vi "Create GB.vi"(5 "Max # of atoms":i32=9999999, 6 "Edge Duplication Range":dbl=3.0, 7 "Skip cleanup if no subset":bool=TRUE, 8 "Reduce to Repeating":T5={"Slab X"=4.6, "Slab Y"=4.0, "Tolerance (A)"=0.5, "Presorted?"=FALSE}, 9 "Min Seperation Distance (A)":dbl=2.0, 10 "Grain Growth and Geometry":T6={"Min Grain 1 Length (A)"=6.0, "Min Grain 2 Length (A)"=6.0, "Max Grain Height (A)"=90.0, "Max Grain Width (A)"=90.0, "Grain 1 Start"=-0.001, "Overlap Region (A)"=0.001}, 11 "Grain Boundary Definition":T7={"Grain 1 Orientation"=[1.0, 0.6019417241891012, 0.029651947654046266], "Grain 2 Orientation"=[1.0, 0.730727623275494, 0.2205637301176], "Twist Angle (Deg)"=0.0, "Translation Vector"=[0.0, 0.0, 0.0]}) -> (0 "GB Data":string[][](array[string])=[["Grain 1, h", "Grain 1, k", "Grain 1, L", "Grain 2, h", "Grain 2, k", "Grain 2, L", "Twist Angle (Deg)", "Translation Tx", "Translation Ty", "Translation Tz", "Tilt Angle (Deg)", "Viewing Angle, h", "Viewing Angle, k", "Viewing Angle, L", "Grain 1 Length (factor)", "Grain 2 Length (factor", "Max Grain Height (A)", "Max Grain Width (A)", "Grain 1 Start", "Overlap Region (A)", "Reduction Slab X", "Reduction Slab Y", "Reduction Tolerance (A)", "Min Atomic Separation Distance", "Edge Duplication Range", "# Atoms"], ["1.000000", "0.601942", "0.029652", "1.000000", "0.730728", "0.220564", "0.000000", "0.000000", "0.000000", "0.000000", "10.024930", "1.000000", "-1.661290", "0.000000", "1.000000", "1.000000", "90.000000", "90.000000", "-0.001000", "0.001000", "4.600000", "4.000000", "0.500000", "2.000000", "3.000000", "12135.000000"]], 1 "Reduced Orthorhombic?":bool, 2 "Reduced Rhombahedral?":bool, 3 "Grain Boundary":T8={"Structure Name"="(0.00) twist [1.000,0.602,0.030] [1.000,0.731,0.221] (0.00,0.00,0.00)T GB", "Lattice vector a"=[270.03, 0.0, 0.0], "Lattice vector b"=[0.0, 270.03, 0.0], "Lattice vector c"=[0.0, 0.0, 6.006], "Atoms Array"=[{"Atom Name"="Cd", "Positions (Direct)"=array6055x3[18165 elements], "Positions (Cartesian)"=array6055x3[18165 elements]}, {"Atom Name"="Te", "Positions (Direct)"=array6080x3[18240 elements], "Positions (Cartesian)"=array6080x3[18240 elements]}], "# of atoms"=12135} {"Atoms Array"."Positions (Cartesian)" format="%#_4f"; "Atoms Array"."Positions (Direct)" format="%#_4f"}, 4 "Ortho and Rhom":T3(array[cluster]) {"Atoms Array"."Positions (Cartesian)" format="%#_4f"; "Atoms Array"."Positions (Direct)" format="%#_4f"})   [LabVIEW 2010]
uses:
  <vilib>/Analysis/NI_AALPro.lvlib
  <vilib>/Analysis/_algsub.llb/Real Vector Norm.vi
  <vilib>/Analysis/NI_AALBase.lvlib
  <vilib>/Analysis/baseanly.llb/A x Vector.vi
  <vilib>/Analysis/baseanly.llb/Real A x B.vi
panel:
  in  "GB Reduction":T1(radio)
  in  "GB Geometry":T2(radio)
  in  "Min Wedge Thickness (A)":dbl=5.0
  out "error out":errorcluster
  out "Original # of atoms":i32=12135
  out "Expected # of Atoms":i32=166
  in  "Integer Tolerance":dbl=0.01
  out "Creation Time":T4={"Time to create primitives"=0, "Time to Grow to Box"=4152, "Time to find subset"=1109, "Time to Cleanup"=1}
  in  "Headers":string[](array[string])=["Grain 1, h", "Grain 1, k", "Grain 1, L", "Grain 2, h", "Grain 2, k", "Grain 2, L", "Twist Angle (Deg)", "Translation Tx", "Translation Ty", "Translation Tz", "Tilt Angle (Deg)", "Viewing Angle, h", "Viewing Angle, k", "Viewing Angle, L", "Grain 1 Length (factor)", "Grain 2 Length (factor", "Max Grain Height (A)", "Max Grain Width (A)", "Grain 1 Start", "Overlap Region (A)", "Reduction Slab X", "Reduction Slab Y", "Reduction Tolerance (A)", "Min Atomic Separation Distance", "Edge Duplication Range", "# Atoms"]
  out "Rhombehedral Atoms":i32=12135
  out "Orthorhombic atoms":i32=12135
  out "Time to Cleanup":u32=1
  out "Time to find subset":u32=1109
  out "Time to Grow to Box":u32=4152
  out "Time to create primitives":u32
  out "Tilt Angle":dbl=10.024929742348679
  out "# of Atoms Removed":i32=28
  out "Repeating Y Length Scale":dbl=13.227303403298492
  out "Repeating X Length Scale":dbl
  out "Mutual Viewing Angle":dbl[](array[numeric])=[1.0, -1.6612903871170226, 0.0]
  in  "Conventional Unit Cell":T8={"Structure Name"="CdTe", "Lattice vector a"=[6.615785553057252, 0.0, 0.0], "Lattice vector b"=[0.0, 6.615785553057252, 0.0], "Lattice vector c"=[0.0, 0.0, 6.615785553057252], "Atoms Array"=[{"Atom Name"="Cd", "Positions (Direct)"=[[0.0, 0.0, 0.0], [0.0, 0.5, 0.5], [0.5, 0.0, 0.5], [0.5, 0.5, 0.0]], "Positions (Cartesian)"=[[0.0, 0.0, 0.0], [0.0, 3.307892776528626, 3.307892776528626], [3.307892776528626, 0.0, 3.307892776528626], [3.307892776528626, 3.307892776528626, 0.0]]}, {"Atom Name"="Te", "Positions (Direct)"=[[0.25, 0.25, 0.25], [0.75, 0.75, 0.25], [0.75, 0.25, 0.75], [0.25, 0.75, 0.75]], "Positions (Cartesian)"=[[1.653946388264313, 1.653946388264313, 1.653946388264313], [4.96183916479294, 4.96183916479294, 1.653946388264313], [4.96183916479294, 1.653946388264313, 4.96183916479294], [1.653946388264313, 4.96183916479294, 4.96183916479294]]}], "# of atoms"=8}
  # "Primitives"
  # "Remove Collisions"
  # "Make into repeating cell"
  # "Grain Growth"
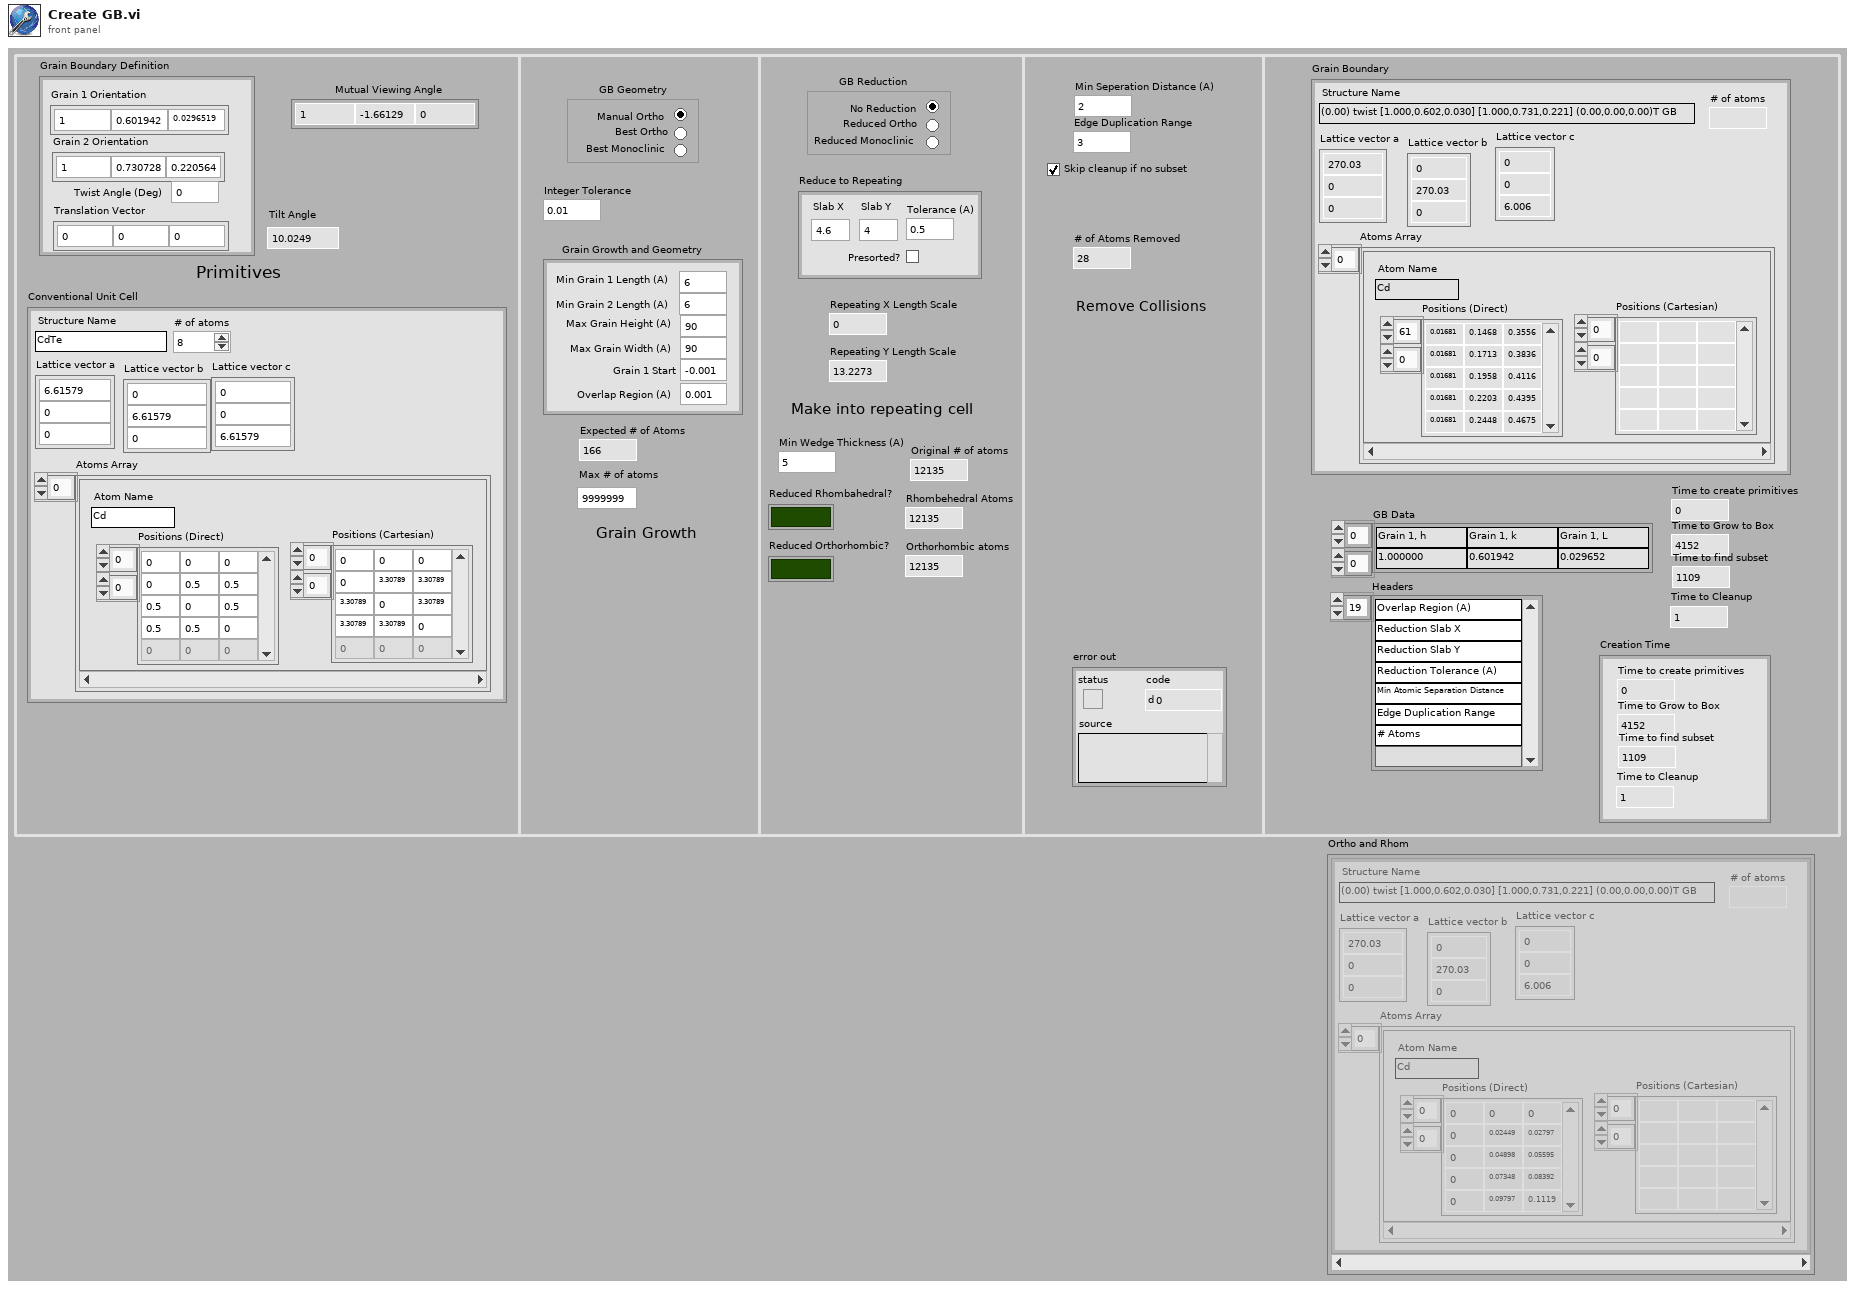
[diagram p1: front panel]
types:
  T1 = enum32{"No Reduction", "Reduced Ortho", "Reduced Monoclinic"}
  T2 = enum32{"Manual Ortho", "Best Ortho", "Best Monoclinic"}
  T3 = cluster{"Structure Name":string, "Lattice vector a":dbl[], "Lattice vector b":dbl[], "Lattice vector c":dbl[], "Atoms Array":cluster{"Atom Name":string, "Positions (Direct)":dbl[][], "Positions (Cartesian)":dbl[][]}[], "# of atoms":i32}[]
  T4 = cluster{"Time to create primitives":u32, "Time to Grow to Box":u32, "Time to find subset":u32, "Time to Cleanup":u32}
  T5 = cluster{"Slab X":dbl, "Slab Y":dbl, "Tolerance (A)":dbl, "Presorted?":bool}
  T6 = cluster{"Min Grain 1 Length (A)":dbl, "Min Grain 2 Length (A)":dbl, "Max Grain Height (A)":dbl, "Max Grain Width (A)":dbl, "Grain 1 Start":dbl, "Overlap Region (A)":dbl}
  T7 = cluster{"Grain 1 Orientation":dbl[], "Grain 2 Orientation":dbl[], "Twist Angle (Deg)":dbl, "Translation Vector":dbl[]}
  T8 = cluster{"Structure Name":string, "Lattice vector a":dbl[], "Lattice vector b":dbl[], "Lattice vector c":dbl[], "Atoms Array":cluster{"Atom Name":string, "Positions (Direct)":dbl[][], "Positions (Cartesian)":dbl[][]}[], "# of atoms":i32}
  T9 = cluster{"Grain 1 Orientation":dbl[], "Grain 2 Orientation":dbl[], "Twist Angle (Deg)":dbl}
  T10 = typedef "NI_Matrix.lvlib/RealMatrix.ctl" = dbl[][]
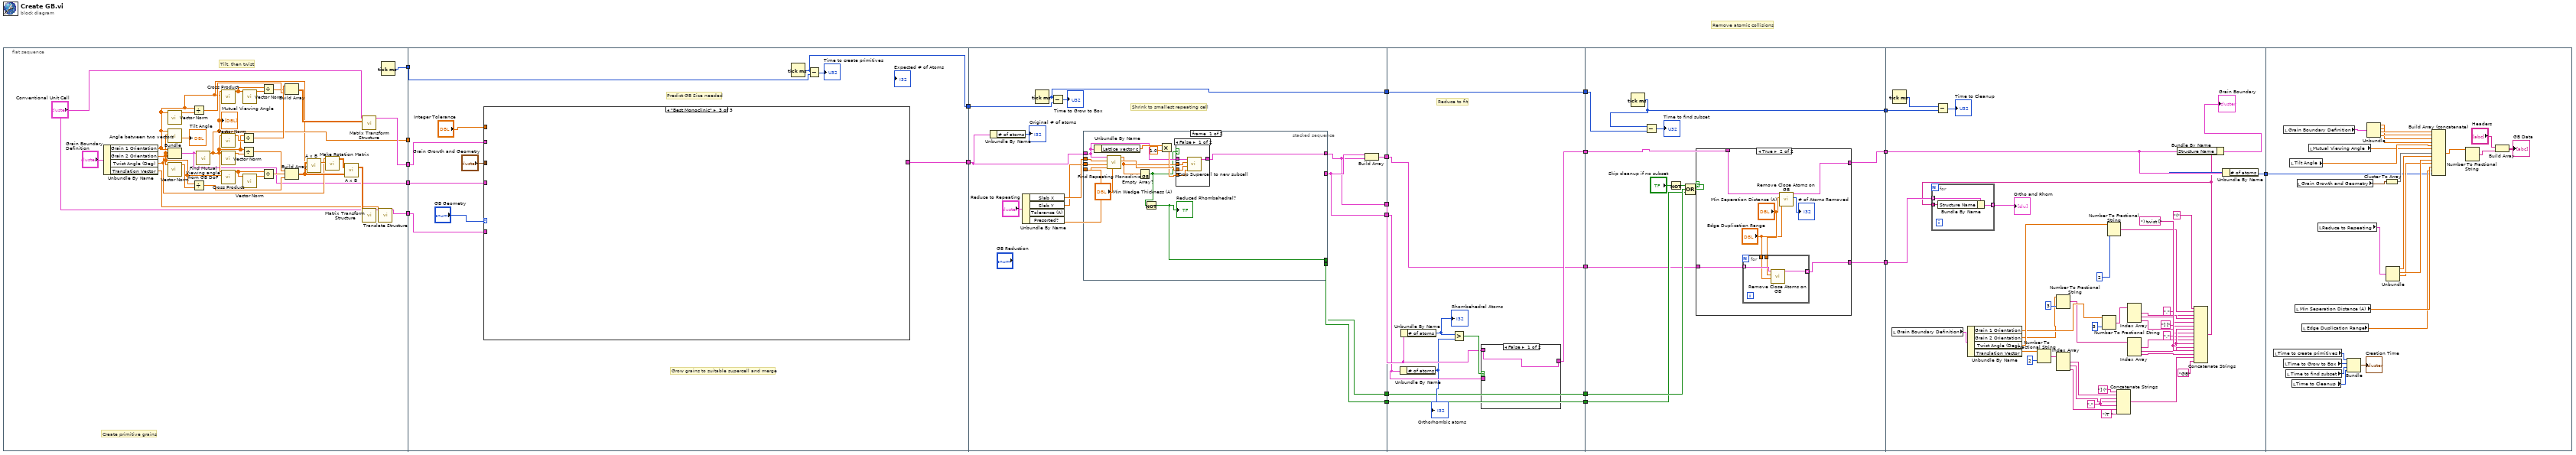
[diagram p0: block diagram]
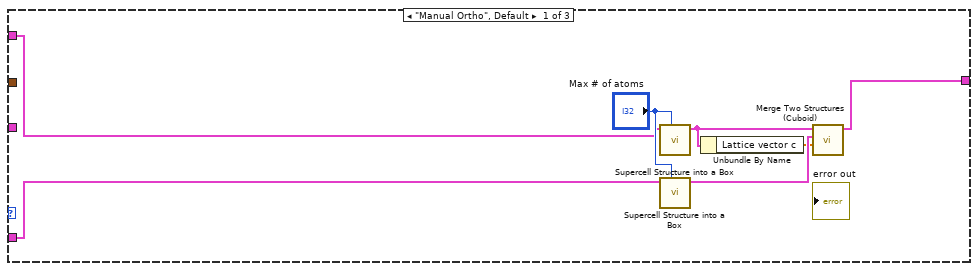
[diagram p2: hidden frame]
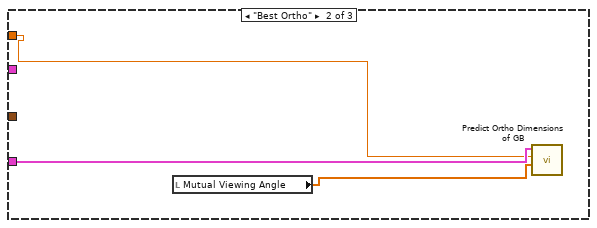
[diagram p3: hidden frame]
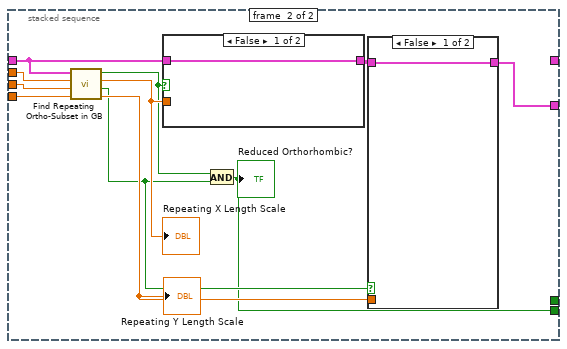
[diagram p5: hidden frame]
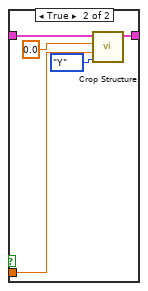
[diagram p6: hidden frame]
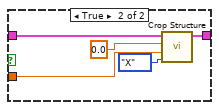
[diagram p7: hidden frame]
diagram:
  # "Remove atomic collisions"
  n1 = flat-sequence {
    tunnel: [w35] -> w10
    tunnel: [w46] -> w9
    tunnel: [w32] -> w8
    tunnel: [w28] -> w7
    tunnel: [w23] -> w1
    tunnel: w10 -> [w57]
    tunnel: w9 -> [w58]
    tunnel: w8 -> [w62]
    tunnel: w7 -> [_]
    tunnel: [w63] -> w3
    tunnel: [w61] -> w2
    tunnel: w1 -> [w55]
    tunnel: [w78] -> w20
    tunnel: [w86] -> w18
    tunnel: [w79] -> w16
    tunnel: [w82] -> w14
    tunnel: [w81] -> w13
    tunnel: [w77] -> w6
    tunnel: w3 -> [w76]
    tunnel: w2 -> [w75]
    tunnel: w20 -> [w138]
    tunnel: [w136] -> w19
    tunnel: w18 -> [w140]
    tunnel: [w140] -> w17
    tunnel: w16 -> [w137]
    tunnel: w14 -> [w132]
    tunnel: w13 -> [w133]
    tunnel: [w133] -> w12
    tunnel: [w132] -> w11
    tunnel: w6 -> [w131]
    tunnel: [w131] -> w5
    tunnel: w19 -> [w154]
    tunnel: [w153] -> w22
    tunnel: w17 -> [w151]
    tunnel: [w150] -> w21
    tunnel: w12 -> [w146]
    tunnel: w11 -> [w145]
    tunnel: w5 -> [w144]
    tunnel: [w143] -> w4
    tunnel: w22 -> [w181]
    tunnel: w21 -> [w182]
    tunnel: [w180] -> w15
    tunnel: w4 -> [w170]
    tunnel: w15 -> [w223]
    frame #0 {
      # "Tilt, then twist"
      # "Create primitive grains"
      n2 = Unbundle By Name("Grain Boundary Definition") -> ("Grain 1 Orientation"=w26:dbl[], "Grain 2 Orientation"=w25:dbl[], "Twist Angle (Deg)"=w24:dbl, "Translation Vector"=w33:dbl[])
      n3 = call-poly <vilib>:"Vector Norm.vi"("Input Vector"=w26) -> ("norm"=w52:dbl)  [unwired: 9 in, 1 out]
      n4 = call "Angle between two vectors.vi"("Vector 2"=w25, "Vector 1"=w26) -> ("Angle (Degrees)"=→"Tilt Angle":dbl)  [unwired: 7 in, 2 out]
      n5 = Bundle("Grain 1 Orientation"=w26, "Grain 2 Orientation"=w25, "Twist Angle (Deg)"=w24) -> (w23:T9)  [unwired: 1 in]
      n6 = call-poly <vilib>:"Vector Norm.vi"("Input Vector"=w25) -> ("norm"=w38:dbl)  [unwired: 9 in, 1 out]
      n7 = Divide(x=w26, y=w52) -> (x/y=w50:dbl[])
      n8 = Divide(x=w25, y=w38) -> (x/y=w40:dbl[])
      n9 = call "Find Mutual Viewing angle from GB DoF.vi"("Grain Boundary Macro DoF"=w23) -> ("Mutual Viewing Angle"=w28:dbl[])  [unwired: 8 in, 2 out]
      "Mutual Viewing Angle" <- w28
      n10 = call <vilib>:"Cross Product.vi"("B Vector"=w26, "A Vector"=w28) -> ("Cross Product"=w48:dbl[])  [unwired: 8 in, 1 out]
      n11 = call-poly <vilib>:"Vector Norm.vi"("Input Vector"=w28) -> ("norm"=w54:dbl)  [unwired: 9 in, 1 out]
      n12 = call-poly <vilib>:"Vector Norm.vi"("Input Vector"=w28) -> ("norm"=w36:dbl)  [unwired: 9 in, 1 out]
      n13 = call <vilib>:"Cross Product.vi"("B Vector"=w25, "A Vector"=w28) -> ("Cross Product"=w41:dbl[])  [unwired: 8 in, 1 out]
      n14 = Divide(x=w28, y=w54) -> (x/y=w51:dbl[])
      n15 = Divide(x=w28, y=w36) -> (x/y=w39:dbl[])
      n16 = call-poly <vilib>:"Vector Norm.vi"("Input Vector"=w48) -> ("norm"=w53:dbl)  [unwired: 9 in, 1 out]
      n17 = call-poly <vilib>:"Vector Norm.vi"("Input Vector"=w41) -> ("norm"=w37:dbl)  [unwired: 9 in, 1 out]
      n18 = Divide(x=w48, y=w53) -> (x/y=w47:dbl[])
      n19 = Divide(x=w41, y=w37) -> (x/y=w45:dbl[])
      n20 = Build Array(w51, w47, w50) -> (w49:T10)
      n21 = Build Array(w39, w45, w40) -> (w30:T10)
      n22 = call-poly <vilib>:"A x B.vi"("Vector"=w26, "A"=w30) -> ("A x Vector"=w29:dbl[])  [unwired: 1 out]
      n23 = call "Make Rotation Matrix.vi"("Rotation Axis"=w29, "Rotation Angle (Degree)"=w24) -> ("Rotation Matrix"=w43:T10)  [unwired: 9 in]
      n24 = call-poly <vilib>:"A x B.vi"("B"=w30, "A"=w43) -> ("A x B"=w42:T10)  [unwired: 1 out]
      n25 = call "Matrix Transform Structure.vi"("Matrix Transform"=w49, "Original Structure"="Conventional Unit Cell") -> ("After Transform"=w46:T8)  [unwired: 9 in]
      n26 = call "Matrix Transform Structure.vi"("Matrix Transform"=w42, "Original Structure"="Conventional Unit Cell") -> ("After Transform"=w44:T8)  [unwired: 9 in]
      n27 = call "Translate Structure.vi"("Translation Vector (Cartesian)"=w33, "Atomic Structure"=w44) -> ("Shifted Structure"=w35:T8)  [unwired: 9 in]
      n28 = Tick Count (ms)() -> (millisecond timer value=w32:u32)
    }
    frame #1 {
      # "Grow grains to suitable supercell and merge"
      # "Predict GB Size needed"
      n29 = case shown="\"Best Monoclinic\"" "GB Geometry" {
        tunnel: [w67 _ _] -> w63
        tunnel: "Grain Growth and Geometry" -> [_ _ _]
        tunnel: w58 -> [w66 _ _]
        tunnel: w57 -> [w65 _ _]
        tunnel: "Integer Tolerance" -> [_ w73 _]
        tunnel: w55 -> [_ w74 _]
        frame "Manual Ortho", Default {
          n30 = call "Supercell Structure into a Box.vi"("Max # of atoms"="Max # of atoms", "Subcrystal"=w66) -> ("Expanded cubic Structure"=w70:T8)  [unwired: 7 in, 2 out]
          n31 = call "Supercell Structure into a Box.vi"("Max # of atoms"="Max # of atoms", "Subcrystal"=w65) -> ("Expanded cubic Structure"=w69:T8)  [unwired: 7 in, 2 out]
          n32 = Unbundle By Name(w70) -> ("Lattice vector c"=w68:dbl[])
          n33 = call "Merge Two Structures (Cuboid).vi"("Translation Vector (1 to 2)"=w68, "Atomic Structure 2"=w69, "Atomic Structure 1"=w70) -> ("Atomic Structure of 1 + 2 by T"=w67:T8)  [unwired: 8 in]
        }
        frame "Best Ortho" {
          n34 = local read "Mutual Viewing Angle"() -> (w72:dbl[])
          n35 = call "Predict Ortho Dimensions of GB.vi"("Mutual Viewing Angle"=w72, "Tolerance"=w73, "Grain Boundary Macro Definition"=w74) -> ()  [unwired: 6 in, 3 out]
        }
        frame "Best Monoclinic" {
        }
      }
      n36 = Tick Count (ms)() -> (millisecond timer value=w61:u32)
      n37 = Subtract(x=w61, y=w62) -> (x-y=→"Time to create primitives":u32)
    }
    frame #2 {
      # "Shrink to smallest repeating cell"
      n38 = Unbundle By Name(w76) -> ("# of atoms"=→"Original # of atoms":i32)
      n39 = Unbundle By Name("Reduce to Repeating") -> ("Slab X"=w85:dbl, "Slab Y"=w84:dbl, "Tolerance (A)"=w83:dbl)  [unwired: 1 out]
      n40 = Tick Count (ms)() -> (millisecond timer value=w86:u32)
      n41 = Subtract(x=w86, y=w75) -> (x-y=→"Time to Grow to Box":u32)
      n42 = stacked-sequence {
        tunnel: [w90 _] -> w78
        tunnel: w85 -> [w96 w118]
        tunnel: w84 -> [w95 w117]
        tunnel: w83 -> [w94 w116]
        tunnel: w76 -> [w97 w115]
        tunnel: [_ w108] -> w79
        tunnel: [_ w109] -> w82
        tunnel: [w91 _] -> w81
        frame #0 {
          n43 = Unbundle By Name(w97) -> ("Lattice vector c"=w99:dbl[])
          n44 = call "Find Repeating Monoclinic GB.vi"("Min Wedge Thickness (A)"="Min Wedge Thickness (A)", "Tolerance (A)"=w94, "Slab Y"=w95, "Slab X"=w96, "Supercell Structure"=w97) -> ("New Lattice Vector b"=w101:dbl[], "New Lattice Vector a"=w93:dbl[])  [unwired: 4 in, 1 out]
          n45 = Empty Array?(array=w93) -> (empty?=w92:bool)
          n46 = Not(x=w92) -> (.not. x?=w91:bool)
          "Reduced Rhombahedral?" <- w91
          n47 = Multiply(x=w99, y=1.0) -> (x*y=w98:dbl[])
          n48 = case shown="False" w92 {
            tunnel: w101 -> [w106 _]
            tunnel: w93 -> [w105 _]
            tunnel: w98 -> [w104 _]
            tunnel: w97 -> [w103 w107]
            tunnel: [w102 w107] -> w90
            frame False {
              n49 = call "Crop Supercell to new subcell.vi"("New Lattice Vector c"=w104, "New Lattice Vector b"=w106, "New Lattice Vector a"=w105, "Supercell Structure"=w103) -> ("Reduced Structure"=w102:T8)  [unwired: 7 in]
            }
            frame True {
            }
          }
        }
        frame #1 {
          n50 = call "Find Repeating Ortho-Subset in GB.vi"("Tolerance (A)"=w116, "Slab Y"=w117, "Slab X"=w118, "Grain Boundary"=w115) -> ("Repeating Y Length Scale"=w112:dbl, "Subset Y found?!"=w110:bool, "Repeating X Length Scale"=w113:dbl, "Subset X found?!"=w111:bool)  [unwired: 4 in]
          "Repeating X Length Scale" <- w113
          "Repeating Y Length Scale" <- w112
          n51 = case shown="False" w111 {
            tunnel: w115 -> [w125 w130]
            tunnel: [w125 w127] -> w114
            tunnel: w113 -> [_ w126]
            frame False {
            }
            frame True {
              n52 = call "Crop Structure.vi"("Cropping Index"=enum16{"X", "Y", "Z"}."X", "Upper Bound Z"=w126, "Lower bound Z"=0.0, "Input Structure"=w130) -> ("Cropped Structure"=w127:T8)  [unwired: 7 in]
            }
          }
          n53 = And(x=w111, y=w110) -> (x .and. y?=w109:bool)
          "Reduced Orthorhombic?" <- w109
          n54 = case shown="False" w110 {
            tunnel: w114 -> [w119 w124]
            tunnel: w112 -> [_ w122]
            tunnel: [w119 w120] -> w108
            frame False {
            }
            frame True {
              n55 = call "Crop Structure.vi"("Cropping Index"=enum16{"X", "Y", "Z"}."Y", "Upper Bound Z"=w122, "Lower bound Z"=0.0, "Input Structure"=w124) -> ("Cropped Structure"=w120:T8)  [unwired: 7 in]
            }
          }
        }
      }
      n56 = Build Array(w79, w78) -> (w77:T3)
    }
    frame #3 {
      # "Reduce to fit"
      n57 = Unbundle By Name(w137) -> ("# of atoms"=w134:i32)
      "Orthorhombic atoms" <- w134
      n58 = Unbundle By Name(w138) -> ("# of atoms"=w135:i32)
      "Rhombehedral Atoms" <- w135
      n59 = Greater?(x=w135, y=w134) -> (0:w139:bool)
      n60 = case shown="False" w139 {
        tunnel: [w141 w142] -> w136
        tunnel: w138 -> [w141 _]
        tunnel: w137 -> [_ w142]
        frame False {
        }
        frame True {
        }
      }
    }
    frame #4 {
      n61 = Tick Count (ms)() -> (millisecond timer value=w150:u32)
      n62 = Subtract(x=w150, y=w151) -> (x-y=→"Time to find subset":u32)
      n63 = Not(x="Skip cleanup if no subset") -> (.not. x?=w148:bool)
      n64 = Compound Arithmetic op=OR(w148, w146, w145) -> (w147:bool)
      n65 = case shown="True" w147 {
        tunnel: w154 -> [w156 w162]
        tunnel: [w156 w161] -> w153
        tunnel: w144 -> [w155 w160]
        tunnel: [w155 w157] -> w143
        frame False {
        }
        frame True {
          n66 = for {
            tunnel: w160 -> [w167] mode=indexing
            tunnel: [w166] -> w157 mode=indexing
            tunnel: "Min Seperation Distance (A)" -> [w165]
            tunnel: "Edge Duplication Range" -> [w164]
            n67 = call "Remove Close Atoms on GB.vi"("Edge Duplication Range"=w164, "Minimally Allowable Distance (A)"=w165, "Structure"=w167) -> ("Structure with atoms removed"=w166:T8)  [unwired: 7 in, 1 out]
          }
          n68 = call "Remove Close Atoms on GB.vi"("Edge Duplication Range"="Edge Duplication Range", "Minimally Allowable Distance (A)"="Min Seperation Distance (A)", "Structure"=w162) -> ("# of Atoms Removed"=→"# of Atoms Removed":i32, "Structure with atoms removed"=w161:T8)  [unwired: 7 in]
        }
      }
    }
    frame #5 {
      w203 = "," ("string")
      w196 = "," ("string")
      n69 = local read "Grain Boundary Definition"() -> (w206:T7)
      n70 = Tick Count (ms)() -> (millisecond timer value=w183:u32)
      n71 = Subtract(x=w183, y=w182) -> (x-y=→"Time to Cleanup":u32)
      n72 = Unbundle By Name(w206) -> ("Grain 1 Orientation"=w177:dbl[], "Grain 2 Orientation"=w174:dbl[], "Twist Angle (Deg)"=w207:dbl, "Translation Vector"=w208:dbl[])
      n73 = Number To Fractional String(number=w208, precision (6)=i16 2) -> (F-format string=w199:string[])  [unwired: 2 in]
      n74 = Number To Fractional String(number=w174, precision (6)=i16 3) -> (F-format string=w173:string[])  [unwired: 2 in]
      n75 = Index Array(array=w199) -> (element #1=w200:string, element #2=w202:string, element #3=w204:string)  [unwired: 3 in]
      n76 = Number To Fractional String(number=w177, precision (6)=i16 3) -> (F-format string=w176:string[])  [unwired: 2 in]
      n77 = Number To Fractional String(number=w207, precision (6)=i16 2) -> (F-format string=w187:string)  [unwired: 2 in]
      n78 = Concatenate Strings("] (" ("string"), w200, w203, w202, w203, w204, ")T " ("string")) -> (w172:string)
      n79 = Index Array(array=w176) -> (element #1=w189:string, element #2=w191:string, element #3=w192:string)  [unwired: 3 in]
      n80 = Index Array(array=w173) -> (element #1=w194:string, element #2=w195:string, element #3=w197:string)  [unwired: 3 in]
      n81 = Concatenate Strings("(" ("string"), w187, ") twist [" ("string"), w189, "," ("string"), w191, w196, w192, "] [" ("string"), w194, w196, w195, w196, w197, w172, "GB" ("string")) -> (w169:string)
      n82 = for {
        tunnel: w170 -> [w211] mode=indexing
        tunnel: w169 -> [w210]
        tunnel: [w209] -> w168 mode=indexing
        n83 = Bundle By Name(cluster=w211, "Structure Name"=w210) -> (w209:T8)
      }
      "Ortho and Rhom" <- w168
      n84 = Bundle By Name(cluster=w181, "Structure Name"=w169) -> (→"Grain Boundary":T8)
      n85 = Unbundle By Name(w181) -> ("# of atoms"=w180:i32)
    }
    frame #6 {
      n86 = local read "Time to create primitives"() -> (w215:u32)
      n87 = local read "Time to Grow to Box"() -> (w214:u32)
      n88 = local read "Grain Boundary Definition"() -> (w236:T7)
      n89 = local read "Time to find subset"() -> (w213:u32)
      n90 = local read "Tilt Angle"() -> (w219:dbl)
      n91 = local read "Time to Cleanup"() -> (w216:u32)
      n92 = local read "Min Seperation Distance (A)"() -> (w225:dbl)
      n93 = local read "Grain Growth and Geometry"() -> (w231:T6)
      n94 = local read "Edge Duplication Range"() -> (w224:dbl)
      n95 = local read "Mutual Viewing Angle"() -> (w218:dbl[])
      n96 = local read "Reduce to Repeating"() -> (w229:T5)
      n97 = Bundle("Time to create primitives"=w215, "Time to Grow to Box"=w214, "Time to find subset"=w213, "Time to Cleanup"=w216) -> (→"Creation Time":T4)  [unwired: 1 in]
      n98 = Unbundle(w236) -> ("Grain 1 Orientation"=w235:dbl[], "Grain 2 Orientation"=w234:dbl[], "Twist Angle (Deg)"=w233:dbl, "Translation Vector"=w232:dbl[])
      n99 = Cluster To Array(cluster=w231) -> (array=w230:dbl[])
      n100 = Unbundle(w229) -> ("Slab X"=w228:dbl, "Slab Y"=w227:dbl, "Tolerance (A)"=w226:dbl)  [unwired: 1 out]
      n101 = Build Array (concatenate)(w235, w234, w233, w232, w219, w218, w230, w228, w227, w226, w225, w224, w223) -> (w222:dbl[])
      n102 = Number To Fractional String(number=w222) -> (F-format string=w221:string[])  [unwired: 3 in]
      n103 = Build Array("Headers", w221) -> (→"GB Data":string[][])
    }
  }
